vi "set_gate_valve_state (SubVI).vi"(5 "transition_time":dbl=5.0 format="%#_13g", 7 "hold_time":dbl=3.0 format="%#_13g", 8 "error in":errorcluster, 10 "operation":u16(ring)=1 items=["actuate_open", "actuate_closed"], 11 "gate_valve_drives":tag="Dev3/Port0/Line1,Dev3/Port0/Line7") -> (0 "error out":errorcluster)   [LabVIEW 2022 SP3]
uses:
  <vilib>/DAQmx/write.llb/DAQmx Write (Digital 1D Bool NChan 1Samp 1Line).vi
  <vilib>/DAQmx/create/channels.llb/DAQmx Create Channel (DO-Digital Output).vi
  <vilib>/DAQmx/miscellaneous.llb/DAQmx Fill In Error Info.vi
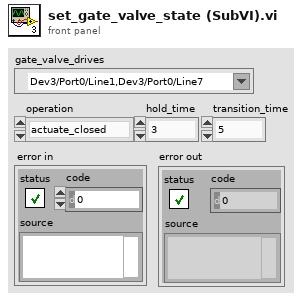
[diagram p1: front panel]
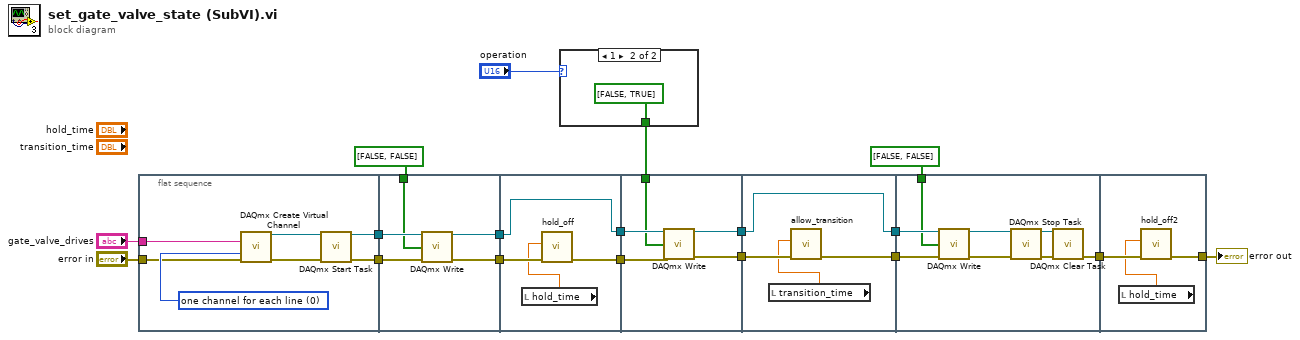
[diagram p0: block diagram]
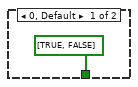
[diagram p2: hidden frame]
diagram:
  n1 = flat-sequence {
    tunnel: "gate_valve_drives" -> [w24]
    tunnel: [w22] -> w18
    tunnel: [w21] -> w17
    tunnel: "error in" -> [w19]
    tunnel: w18 -> [w30]
    tunnel: w17 -> [w29]
    tunnel: [w28] -> w16
    tunnel: [w27] -> w14
    tunnel: bool[] [FALSE, FALSE] ("data") -> [w26]
    tunnel: w16 -> [w34]
    tunnel: [w33] -> w15
    tunnel: w14 -> [w32]
    tunnel: [w32] -> w13
    tunnel: w15 -> [w38]
    tunnel: w13 -> [w39]
    tunnel: [w37] -> w12
    tunnel: [w36] -> w11
    tunnel: w7 -> [w35]
    tunnel: w12 -> [w43]
    tunnel: w11 -> [w41]
    tunnel: [w42] -> w10
    tunnel: [w41] -> w9
    tunnel: w10 -> [w51]
    tunnel: w9 -> [w50]
    tunnel: bool[] [FALSE, FALSE] ("data") -> [w45]
    tunnel: [w44] -> w1
    tunnel: [w53] -> w3
    tunnel: w1 -> [w54]
    frame #0 {
      w20 = 0 items=["one channel for each line", "one channel for all lines"] ("line grouping")
      n2 = call-poly <vilib>:"DAQmx Create Virtual Channel.vi"("lines"=w24, "line grouping"=w20, "error in"=w19) -> ("task out"=w25:refnum<k21>, "error out"=w23:errorcluster)  [unwired: 11 in]
      n3 = call <vilib>:"DAQmx Start Task.vi"("task/channels in"=w25, "error in"=w23) -> ("task out"=w21:refnum<k21>, "error out"=w22:errorcluster)  [unwired: 12 in]
    }
    frame #1 {
      n4 = call-poly <vilib>:"DAQmx Write.vi"("task/channels in"=w29, "data"=w26, "error in"=w30) -> ("task out"=w27:refnum<k21>, "error out"=w28:errorcluster)  [unwired: 10 in, 1 out]
    }
    frame #2 {
      n5 = local read "hold_time"() -> (w31:dbl)
      n6 = call "hold_off"("error in (no error)"=w34, "Delay Time (s)"=w31) -> ("error out"=w33:errorcluster)  [unwired: 9 in]
    }
    frame #3 {
      n7 = call-poly <vilib>:"DAQmx Write.vi"("task/channels in"=w39, "data"=w35, "error in"=w38) -> ("task out"=w36:refnum<k21>, "error out"=w37:errorcluster)  [unwired: 10 in, 1 out]
    }
    frame #4 {
      n8 = local read "transition_time"() -> (w40:dbl)
      n9 = call "allow_transition"("error in (no error)"=w43, "Delay Time (s)"=w40) -> ("error out"=w42:errorcluster)  [unwired: 9 in]
    }
    frame #5 {
      n10 = call-poly <vilib>:"DAQmx Write.vi"("task/channels in"=w50, "data"=w45, "error in"=w51) -> ("task out"=w47:refnum<k21>, "error out"=w46:errorcluster)  [unwired: 10 in, 1 out]
      n11 = call <vilib>:"DAQmx Stop Task.vi"("task/channels in"=w47, "error in"=w46) -> ("task out"=w49:refnum<k21>, "error out"=w48:errorcluster)  [unwired: 12 in]
      n12 = call <vilib>:"DAQmx Clear Task.vi"("task in"=w49, "error in"=w48) -> ("error out"=w44:errorcluster)  [unwired: 13 in]
    }
    frame #6 {
      n13 = local read "hold_time"() -> (w52:dbl)
      n14 = call "hold_off2"("error in (no error)"=w54, "Delay Time (s)"=w52) -> ("error out"=w53:errorcluster)  [unwired: 9 in]
    }
  }
  n15 = case shown="1" "operation" {
    tunnel: [bool[] [TRUE, FALSE] ("data") bool[] [FALSE, TRUE] ("data")] -> w7
    frame 0, Default {
    }
    frame 1 {
    }
  }
  "error out" <- w3
